vi "Main.vi"() -> ()   [LabVIEW 2013]
uses:
  <vilib>/myRIO/Instrument Drivers/Onboard IO/DIO/vis/Smart Open.vi
  <vilib>/myRIO/Instrument Drivers/Onboard IO/DIO/vis/Read.vi
  <vilib>/myRIO/Common/Instrument Driver Framework/myRIO v1.0/UART/vis/myRIO v1.0 Close UART.vi
  <vilib>/myRIO/Instrument Drivers/Onboard IO/DIO/vis/Open.vi
  <vilib>/myRIO/Common/Instrument Driver Framework/myRIO v1.0/DIO/vis/myRIO v1.1 Open DIO.vi
  <vilib>/myRIO/Common/Instrument Driver Framework/Utilities/vis/Validate Channels.vi
  <vilib>/myRIO/Common/Instrument Driver Framework/myRIO v1.0/DIO/vis/myRIO v1.0 Reserve DIO.vi
  <vilib>/myRIO/Common/Instrument Driver Framework/myRIO v1.0/Resource Manager/vis/myRIO v1.0 Reserve Channel List.vi
  <vilib>/myRIO/Common/Instrument Driver Framework/myRIO v1.0/DIO/vis/myRIO v1.0 Build MUX Configuration DIO.vi
  <vilib>/myRIO/Common/Instrument Driver Framework/myRIO v1.0/Resource Manager/vis/myRIO v1.0 Reserve Channel.vi
  <vilib>/myRIO/Common/Instrument Driver Framework/myRIO v1.0/Resource Manager/vis/myRIO v1.0 Unreserve Channel.vi
  <vilib>/myRIO/Common/Instrument Driver Framework/myRIO v1.0/Resource Manager/vis/myRIO v1.0 Create Configuration List.vi
  <vilib>/myRIO/Common/Instrument Driver Framework/myRIO v1.0/Resource Manager/vis/myRIO v1.0 Build Mutex Name.vi
  <vilib>/Instr/_visa.llb/VISA Configure Serial Port (Instr).vi
  <vilib>/myRIO/Common/Instrument Driver Framework/myRIO v1.0/myRIO v1.1 Open.vi
  <vilib>/Utility/VariantDataType/GetNumericInfo.vi
  <vilib>/Utility/error.llb/Error Cluster From Error Code.vi
  <vilib>/myRIO/Common/Instrument Driver Framework/Utilities/vis/IO Manager.vi
  <vilib>/myRIO/Common/Instrument Driver Framework/Utilities/vis/Configuration Manager.vi
  <vilib>/myRIO/Common/Instrument Driver Framework/myRIO v1.0/Resource Manager/vis/myRIO v1.0 Configure IO.vi
  <vilib>/myRIO/Common/Instrument Driver Framework/myRIO v1.0/myRIO v1.0 Close.vi
  <vilib>/myRIO/Common/Instrument Driver Framework/myRIO v1.0/DIO/vis/myRIO v1.0 Read DIO.vi
  <vilib>/myRIO/Common/Instrument Driver Framework/Utilities/vis/FPGA Ref Manager.vi
  <vilib>/myRIO/Common/Instrument Driver Framework/myRIO v1.0/myRIO v1.0 Reset FPGA.vi
  <vilib>/myRIO/Instrument Drivers/Utilities/Utilities.lvlib
panel:
  out "data string":string
  out "RFID tag bytes":u8[](array[numeric]) format="%02x"
  out "tag detected":bool
  in  "[ESC]":bool
  # "RFID demo"
  # "STX"
  # "Data"
  # "Checksum"
  # "CR / LF"
  # "ETX"
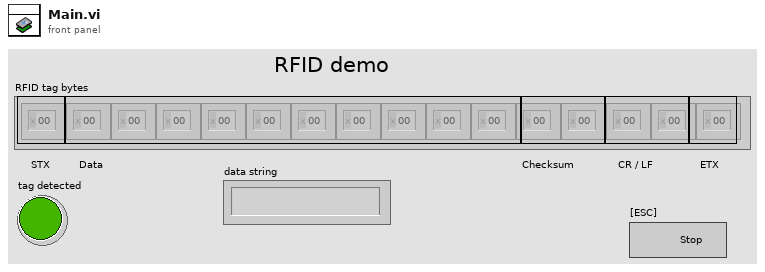
[diagram p1: front panel]
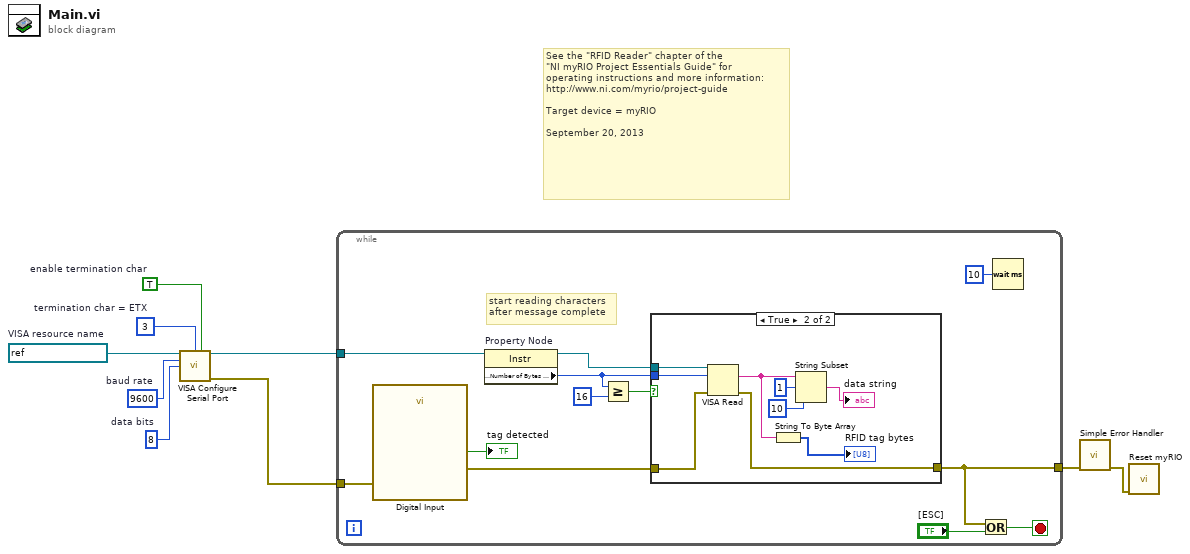
[diagram p0: block diagram]
diagram:
  w2 = TRUE  # enable termination char
  w3 = u16 8  # data bits
  w4 = u32 9600  # baud rate
  w6 = u8 3  # termination char = ETX
  w7 = refnum<visa-resource-name> "ASRL2::INSTR"  # VISA resource name
  # "See the \"RFID Reader\" chapter of the\n\"NI myRIO Project Essentials Guide\" for\noperating instructions and more information: \nhttp://www.ni.com/myrio/project-guide\n\nTarget device = myRIO\n\nSeptember 20, 2013"
  n1 = call-poly "VISA Configure Serial Port"("VISA resource name"=w7, "termination char\n(0xA = '\\n' = LF)"=w6, "Enable Termination\nChar (T)"=w2, "baud rate (9600)"=w4, "data bits (8)"=w3) -> ("VISA resource name out"=w5:refnum<visa-resource-name>, "error out"=w1:errorcluster)  [unwired: 9 in]
  n2 = while {
    tunnel: [w16] -> w8
    tunnel: w5 -> [w10]
    tunnel: w1 -> [w11]
    stop <- w18 stop-if-true
    # "start reading characters\nafter message complete"
    n3 = call "Digital Input"("error in (no error)"=w11) -> ("B/DIO0 (Pin 11)"=→"tag detected":bool, "error out"=w17:errorcluster)  [unwired: 25 in]
    n4 = property on="Property Node" class="Instr"(reference=w10) -> (reference out=w15:refnum<visa-resource-name>, "Serial Settings:Number of Bytes at Serial Port"=w13:u32)  [unwired: 1 in, 1 out]
    n5 = Greater Or Equal?(x=w13, y=u32 16) -> (x >= y?=w14:bool)
    n6 = case shown="True" w14 {
      tunnel: w17 -> [w22 w31]
      tunnel: [w22 w30] -> w16
      tunnel: w15 -> [_ w29]
      tunnel: w13 -> [_ w26]
      frame False {
      }
      frame True {
        n7 = VISA Read(VISA resource name=w29, byte count=w26, error in (no error)=w31) -> (read buffer=w23:string, error out=w30:errorcluster)  [unwired: 2 out]
        n8 = String To Byte Array(string=w23) -> (unsigned byte array=→"RFID tag bytes":u8[])
        n9 = String Subset(string=w23, offset (0)=1, length (rest)=10 ("length (rest)")) -> (substring=→"data string":string)
      }
    }
    n10 = Or(x=w16, y="[ESC]") -> (x .or. y?=w18:bool)
    n11 = Wait (ms)(milliseconds to wait=u32 10) -> ()  [unwired: 1 out]
  }
  n12 = call <vilib>:"Simple Error Handler.vi"("error in (no error)"=w8) -> ("error out"=w9:errorcluster)  [unwired: 4 in, 4 out]
  n13 = call <vilib>:"Reset myRIO.vi"("error in (no error)"=w9) -> ()  [unwired: 10 in, 1 out]
